vi "PS35_Connect.vi"(0 "Interface":i32, 1 "Control unit ID":i32=1 min=1 max=20, 5 "par1":i32=1, 7 "par2":i32=9600, 9 "par3":i32, 11 "error in (no error)":errorcluster, 12 "par4":i32, 13 "par5":i32, 14 "par6":i32 min=0 max=1000) -> (10 "error out":errorcluster)   [LabVIEW 2020]
doc: "PS35_Connect.vi, created: 03.03.2009 alex; last change: 22.10.2019 alex;\n\n<B>FUNCTION:</B> \n\nOpen interface and connect to PS 35.\n*Serial interface (communication via USB or serial port)*\nThe application software can access this interface in the same way as \nit would access a standard serial port (COM). The parameters for Baudrate, \nParity, Databits and Stopbits are predefined (9600, no parity, 8 databits, 1 stopbit).\nThe software handshake character is CR.\n*Ethernet interface (communication via Com-Server)*\nAs Com-Server the OWIS software tool \"OWISerialServer.exe\" may be used\n(..\\OWISoft\\Application\\system). Alternatively, you can use other commercial\nproducts (hardware/software). The application software can access this interface\nvia Windows TCP socket: \nspecial communication for OWIS software (command + delay);\ncommon communication for other software/hardware (command).\nThe software handshake character is CR.\n----------------------------------------------------------------------------------------\n<B>INPUT:</B>\n[I32] <B>Control unit ID:</B> control unit index 1-10. (Default=1, Range=1...20) \n11...20 - debug mode\n1...10 - standard mode\n[I32] <B>Interface:</B> define interface. (Default=0)\nUSB or serial port (=0)\n[I32] <B>par1:</B> define COM port. (Default=1 - COM1, Range=0...255) \n[I32] <B>par2:</B> define request mode for communication. (Default=9600) \n115200 - fast read (all bytes, fast check)\n19200 - fast read (all bytes, slow check)\n9600* - standard read (byte-by-byte)\n[I32] <B>par3:</B> define delay value (=20+x) for serial communication. \n(Default=20 ms) \n[I32] <B>par4:</B> system value. (Default=0) \n10 - without check\n0* - with check (firmware, terminal mode, clear error)\n[I32] <B>par5:</B> system value. (Default=0) \n10 - with port flush\n0* - without port flush\n[I32] <B>par6:</B> system value. (Default=0) \n5 - reconnect for every message\n0* - without reconnect\nEthernet interface + delay in ms (=20+x)\n[I32] <B>par1:</B> define ip address (block 1). (Default=0, Range=0...255) \n[I32] <B>par2:</B> define ip address (block 2). (Default=0, Range=0...255) \n[I32] <B>par3:</B> define ip address (block 3). (Default=0, Range=0...255) \n[I32] <B>par4:</B> define ip address (block 4). (Default=0, Range=0...255) \n[I32] <B>par5:</B> define port number. (Default=1200) \n[I32] <B>par6:</B> system value. (Default=0) \n5 - activate reconnect for every message (option 1)\n6 - activate common communication for other software/hardware (option 2)\n7 - activate both options (1 & 2)\n0* - deactivate both options (1 & 2)\n- without reconnect\n- special communication for OWIS software\n10...20 - without check\n0* - with check\n[CLU] <B>error in</B>\n* - all other values.\n----------------------------------------------------------------------------------------\n<B>OUTPUT:</B>\n[CLU] <B>error out</B>\n0 - no error\n1 - function error (invalid parameters),\n3 - invalid serial port (port is not found),\n4 - access denied (port is busy),\n5 - no response from control unit (check cable, connection or reset control unit),\n9 - no connection to tcp/ip socket.\n----------------------------------------------------------------------------------------\n<B>SUB-VIs:</B>\n----------------------------------------------------------------------------------------\n<B>EXT-Calls:</B>\nps35.dll (V2.01)\n----------------------------------------------------------------------------------------"
uses:
  ps35.dll
panel:
  # "Interface:\n0 - serial                 1(+x) - ethernet (+ delay in ms)"
  # "COM port:\n0 - COM0\n1 - COM1\n..........\n255 - COM255"
  # "IP address:\nblock 1 (0...255)"
  # "Baudrate:\n9600\n19200\n38400\n57600\n115200"
  # "IP address:\nblock 2 (0...255)"
  # "IP address:\nblock 3 (0...255)"
  # "Delay:\nin ms"
  # "IP address:\nblock 4 (0...255)"
  # "Network port:\n 1200"
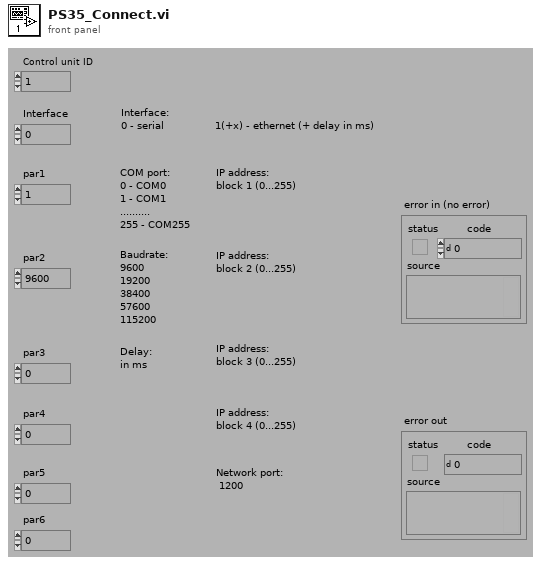
[diagram p1: front panel]
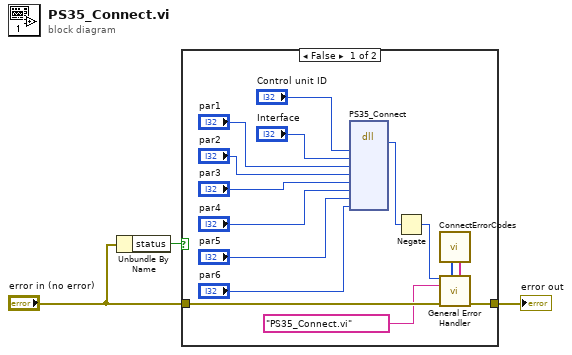
[diagram p0: block diagram]
diagram:
  n1 = Unbundle By Name("error in (no error)") -> ("status"=w1:bool)
  n2 = case shown="False" w1 {
    tunnel: "error in (no error)" -> [w15 w19]
    tunnel: [w17 w19] -> w3
    frame False {
      n3 = dll-call lib="C:/GEECS/Developers Version/source/Device Drivers/OwiSoft/OWISoftOEM/ps35/labview/lv82/ps35.dll" fn="PS35_Connect"("Index"="Control unit ID", "Interface"="Interface", "par1"="par1", "par2"="par2", "par3"="par3", "par4"="par4", "par5"="par5", "par6"="par6") -> ("Rückgabetyp"=w16:i32)  [unwired: 11 in, 2 out]
      n4 = Negate(x=w16) -> (-x=w14:i32)
      n5 = call "ConnectErrorCodes.vi"() -> ("[user-defined codes]"=w5:i32[], "[user-defined descriptions]"=w4:string[])  [unwired: 8 in]
      n6 = call <vilib>:"General Error Handler.vi"("[error code] (0)"=w14, "[user-defined codes]"=w5, "[user-defined descriptions]"=w4, "[error source] (\" \")"="PS35_Connect.vi", "error in (no error)"=w15) -> ("error out"=w17:errorcluster)  [unwired: 6 in, 4 out]
    }
    frame True {
    }
  }
  "error out" <- w3
